vi "Write Charact Result Post Action.vi"(0 "Charact Result Accessor in":refnum<class "Charact Result Accessor.lvclass">, 11 "error in":errorcluster) -> (4 "Charact Result Accessor out":refnum<class "Charact Result Accessor.lvclass">, 15 "error out":errorcluster)   [LabVIEW 2023, in "RFFixtureCharact.RFPM.lvlib" / "Charact Result Accessor.lvclass"]
uses:
  Charact Result Accessor.lvclass
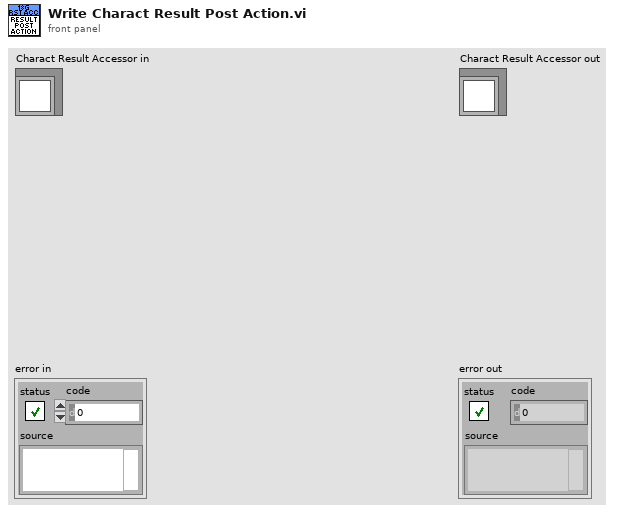
[diagram p1: front panel]
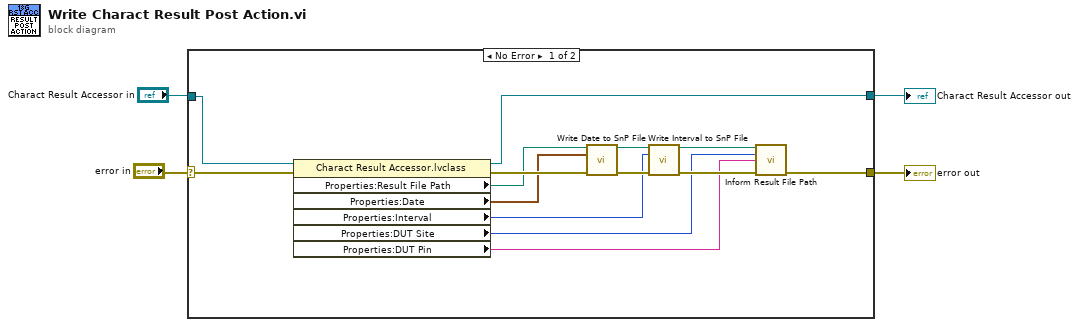
[diagram p0: block diagram]
diagram:
  n1 = case shown="No Error" "error in" {
    selector: "error in" -> [w14 w20]
    tunnel: [w16 w20] -> w2
    tunnel: "Charact Result Accessor in" -> [w15 w19]
    tunnel: [w5 w19] -> w1
    frame No Error {
      n2 = property class="Charact Result Accessor.lvclass"(reference=w15, error in=w14) -> (reference out=w5:refnum<class "Charact Result Accessor.lvclass">, error out=w13:errorcluster, "Properties:Result File Path"=w12:path, "Properties:Date"=w11:timestamp, "Properties:Interval"=w9:i32, "Properties:DUT Site"=w7:i32, "Properties:DUT Pin"=w6:string)
      n3 = call "Write Date to SnP File.vi"("Result File Path In"=w12, "Date"=w11, "error in"=w13) -> ("Result File Path Out"=w10:path, "error out"=w18:errorcluster)  [unwired: 11 in]
      n4 = call "Write Interval to SnP File.vi"("Result File Path In"=w10, "Interval"=w9, "error in"=w18) -> ("Result File Path Out"=w8:path, "error out"=w17:errorcluster)  [unwired: 11 in]
      n5 = call "Inform Result File Path.vi"("Result File Path"=w8, "DUT Site"=w7, "DUT Pin"=w6, "error in"=w17) -> ("error out"=w16:errorcluster)  [unwired: 11 in]
    }
    frame Error {
    }
  }
  "error out" <- w2
  "Charact Result Accessor out" <- w1
